vi "Server_Main Release.vi"(8 "error in":errorcluster) -> (0 "error out":errorcluster)   [LabVIEW 2018, in "Cloud Server.lvlib"]
doc: "進行伺服器主程式的資源釋放。"
uses:
  Cloud Server.lvlib
  Data Def/Server_Error Handle Method.ctl
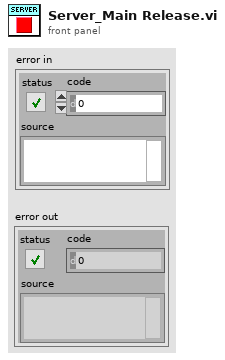
[diagram p1: front panel]
types:
  T1 = typedef "Cloud Server.lvlib/Server_Error Handle Method.ctl" = enum16{"Initialize", "Get Queue Ref.", "Enqueue", "Insert", "Flush", "Release"}
  T2 = typedef "Cloud Server.lvlib/Server_Main Data.ctl" = cluster{"Main VI Ref.":refnum<vi>, "Listener ID":refnum<k5>, "Meta data":T3[], "Main Queue":T5, "User Picture":T6}
  T3 = typedef "stm_MetaElement.ctl" = cluster{"Name":T4}
  T4 = typedef "stm_MetaDataElement.ctl" = string
  T5 = typedef "Cloud Server.lvlib/Server_Main Queue.ctl" = cluster{"Server Write Queue":refnum<queue>, "Main Loop Queue":refnum<queue>}
  T6 = typedef "IMAQ Image.ctl" = refnum<image>
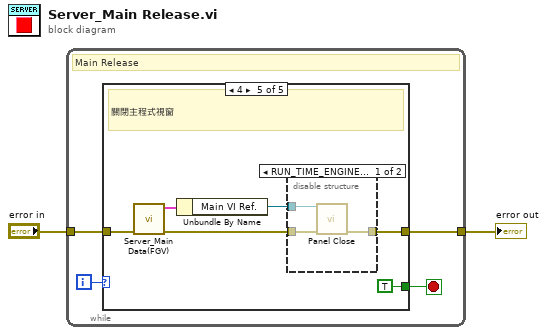
[diagram p0: block diagram]
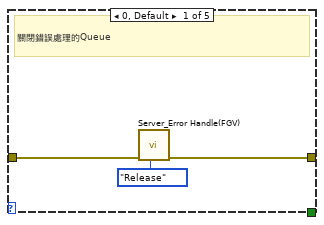
[diagram p2: hidden frame]
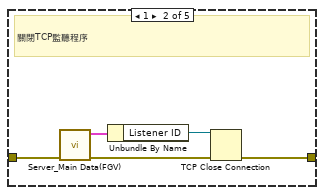
[diagram p3: hidden frame]
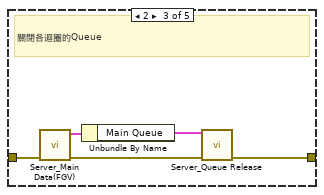
[diagram p4: hidden frame]
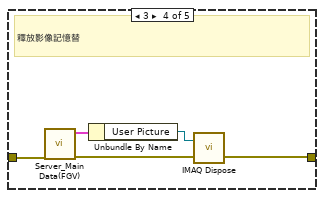
[diagram p5: hidden frame]
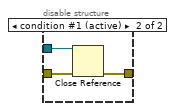
[diagram p6: hidden frame]
diagram:
  n1 = while {
    tunnel: "error in" -> [w5]
    tunnel: [w4] -> w1
    i -> [w6]
    stop <- w3 stop-if-true
    # "Main Release"
    n2 = case shown="4" w6 {
      tunnel: w5 -> [w9 w13 w18 w23 w30]
      tunnel: [w7 w10 w15 w21 w27] -> w4
      tunnel: [_ _ _ _ TRUE] -> w3
      frame 0, Default {
        # "關閉錯誤處理的Queue"
        n3 = call "Server_Error Handle(FGV).vi"("Error Handle Method(Enqueue)"=Server_Error_Handle_Method."Release", "error in"=w9) -> ("error out"=w7:errorcluster)  [unwired: 8 in, 1 out]
      }
      frame 1 {
        # "關閉TCP監聽程序"
        n4 = call "Server_Main Data(FGV).vi"("error in"=w13) -> ("error out"=w12:errorcluster, "Main Data Out"=w14:T2)  [unwired: 9 in]
        n5 = Unbundle By Name(w14) -> ("Listener ID"=w11:refnum<k5>)
        n6 = TCP Close Connection(connection ID=w11, error in (no error)=w12) -> (error out=w10:errorcluster)  [unwired: 1 in, 1 out]
      }
      frame 2 {
        # "關閉各迴圈的Queue"
        n7 = call "Server_Main Data(FGV).vi"("error in"=w18) -> ("error out"=w17:errorcluster, "Main Data Out"=w19:T2)  [unwired: 9 in]
        n8 = Unbundle By Name(w19) -> ("Main Queue"=w16:T5)
        n9 = call "Server_Queue Release.vi"("error in"=w17, "Main Queue"=w16) -> ("error out"=w15:errorcluster)  [unwired: 9 in]
      }
      frame 3 {
        # "釋放影像記憶替"
        n10 = call "Server_Main Data(FGV).vi"("error in"=w23) -> ("error out"=w22:errorcluster, "Main Data Out"=w24:T2)  [unwired: 9 in]
        n11 = Unbundle By Name(w24) -> ("User Picture"=w20:T6)
        n12 = call "IMAQ Dispose"("Image"=w20, "error in (no error)"=w22) -> ("error out"=w21:errorcluster)  [unwired: 4 in]
      }
      frame 4 {
        # "關閉主程式視窗"
        n13 = call "Server_Main Data(FGV).vi"("error in"=w30) -> ("error out"=w28:errorcluster, "Main Data Out"=w29:T2)  [unwired: 9 in]
        n14 = Unbundle By Name(w29) -> ("Main VI Ref."=w26:refnum<vi>)
        n15 = disable-structure shown="RUN_TIME_ENGINE==True, Default" {
          disable-tunnel: w28 -> [w33 w35]
          disable-tunnel: [w32 w36] -> w27
          disable-tunnel: w26 -> [w31 w34]
          frame condition #0 {
            n16 = call "Panel Close.vi"("error in"=w33, "VI Reference"=w31) -> ("error out"=w32:errorcluster)  [unwired: 9 in]
          }
          frame condition #1 (active) {
            n17 = Close Reference(reference=w34, error in (no error)=w35) -> (error out=w36:errorcluster)
          }
        }
      }
    }
  }
  "error out" <- w1
